vi "SensorInterface_API_Close.vi"(5 "Who send this":T1, 8 "error in (no error)":errorcluster, 10 "DataToSend":variant) -> (0 "error out":errorcluster)   [LabVIEW 2013]
doc: "This is part of API."
uses:
  General/Controls/#TD_General_CommunicationQueueStates_Enum.ctl
  Private controls/#TD_SensorInterface_ModuleStates_Enum.ctl
  Private controls/#TD_SensorInterface_ModuleData_Cluster.ctl
  General/Controls/#TD_General_FromWho_Enum.ctl
panel:
  # "INPUT"
  # "OUTPUT"
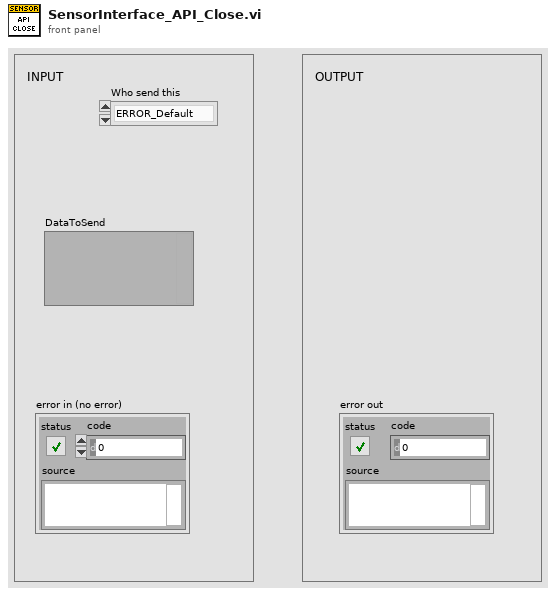
[diagram p1: front panel]
types:
  T1 = typedef "#TD_General_FromWho_Enum.ctl" = enum16{"ERROR_Default", "UserConsole", "DisplayConsole", "SensorInterface", "Controller", "Database", "Timing", "ErrorHandling"}
  T2 = typedef "#TD_General_CommunicationQueueStates_Enum.ctl" = enum16{"ERROR_Default", "Obtain", "GetRef", "Enqueue", "EnqueueAtOpp", "GetStatus", "Release"}
  T3 = typedef "#TD_SensorInterface_ModuleData_Cluster.ctl" = cluster{"Action":T4, "Data":variant}
  T4 = typedef "#TD_SensorInterface_ModuleStates_Enum.ctl" = enum16{"ERROR_Default", "Init", "Close", "ErrorHandling", "DepositReceived", "FundsDispensed"}
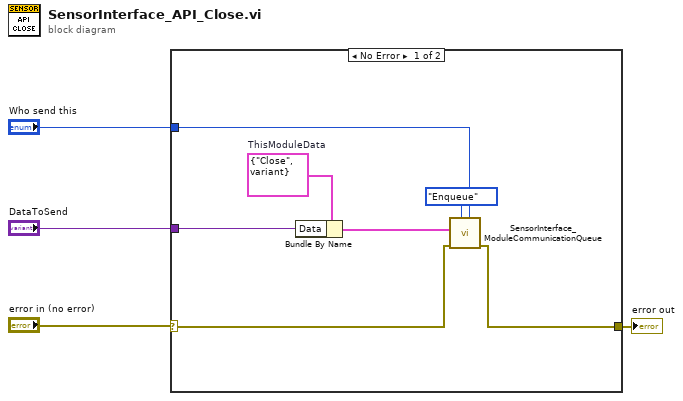
[diagram p0: block diagram]
diagram:
  n1 = case shown="No Error" "error in (no error)" {
    selector: "error in (no error)" -> [w10 w12]
    tunnel: [w9 w12] -> w4
    tunnel: "DataToSend" -> [w6 _]
    tunnel: "Who send this" -> [w5 _]
    frame No Error {
      w8 = T3 {"Action"=enum."Close", "Data"=variant}  # ThisModuleData
      n2 = Bundle By Name(cluster=w8, "Data"=w6) -> (w7:T3)
      n3 = call "SensorInterface_ModuleCommunicationQueue.vi"("Who send this"=w5, "Action"=#TD_General_CommunicationQueueStates_Enum."Enqueue", "error in (no error)"=w10, "ModuleData"=w7) -> ("error out"=w9:errorcluster)  [unwired: 5 in, 2 out]
    }
    frame Error {
    }
  }
  "error out" <- w4
